vi "Configure Hold.vi"(8 "error in (no error)":errorcluster, 9 "Threshold (1:0.1%)":i32(ring)=1 items=["0.01%", "0.1%", "1%", "10%"], 10 "Enable Hold Measurement (F: Disable)":bool, 11 "VISA resource name":refnum<visa-resource-name>) -> (0 "error out":errorcluster, 3 "VISA resource name out":refnum<visa-resource-name>)   [LabVIEW 2021, in "GWInstek  GDM8351.lvlib"]
doc: "Configures the hold measurement and sets the threshold."
uses:
  <instrlib>/GWInstek  GDM8351/GWInstek  GDM8351.lvlib
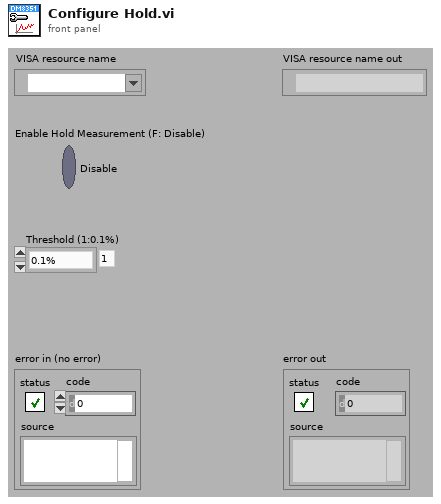
[diagram p1: front panel]
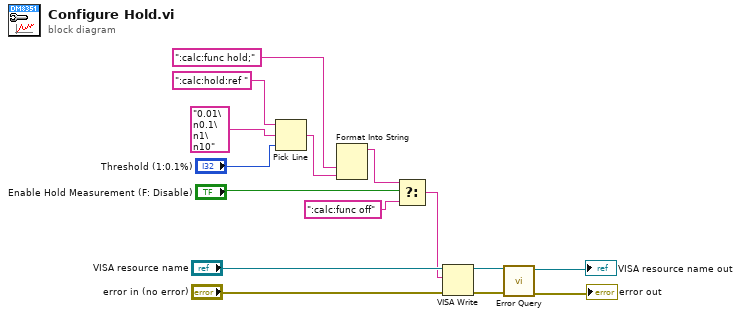
[diagram p0: block diagram]
diagram:
  n1 = Pick Line(string ("")=":calc:hold:ref ", multi-line string="0.01\n0.1\n1\n10", line index="Threshold (1:0.1%)") -> (output string=w5:string)
  n2 = Format Into String(":calc:func hold;" ("string (\"\")"), w5) -> (resulting string=w1:string)  [unwired: 3 in, 1 out]
  n3 = Select(t=w1, s="Enable Hold Measurement (F: Disable)", f=":calc:func off") -> (s? t:f=w2:string)
  n4 = VISA Write(VISA resource name="VISA resource name", write buffer=w2, error in (no error)="error in (no error)") -> (VISA resource name out=w13:refnum<visa-resource-name>, error out=w12:errorcluster)  [unwired: 1 out]
  n5 = call <instrlib>:"Error Query.vi"("error in (no error)"=w12, "VISA resource name"=w13) -> ("error out"=→"error out":errorcluster, "VISA resource name out"=→"VISA resource name out":refnum<visa-resource-name>)  [unwired: 6 in, 2 out]
